vi "Update Command.vi"(6 "Time":dbl, 8 "error in (no error)":errorcluster, 11 "2WayValve in":refnum<class "2WayValveH.lvclass">) -> (0 "error out":errorcluster, 3 "2WayValve out":refnum<class "2WayValveH.lvclass">)   [LabVIEW 2020, in "VolatusGUIElements.lvlib" / "2WayValveH.lvclass"]
uses:
  2WayValveH.lvclass
  2WayValveH.lvclass/2WayValveH.ctl
  lv-vecto/Vecto/Channel/Channel.lvclass/Channel.ctl
  lv-vecto/Vecto/Group/Value by Index.vi
  lv-vecto/Vecto/Channel/Channel.lvclass
  lv-vecto/Vecto/Vecto.lvlib
  VolatusGUIElements.lvlib
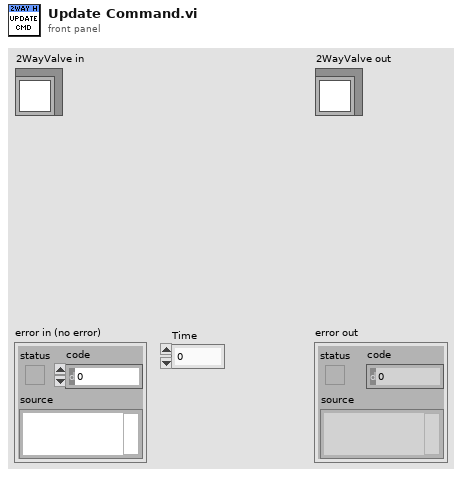
[diagram p1: front panel]
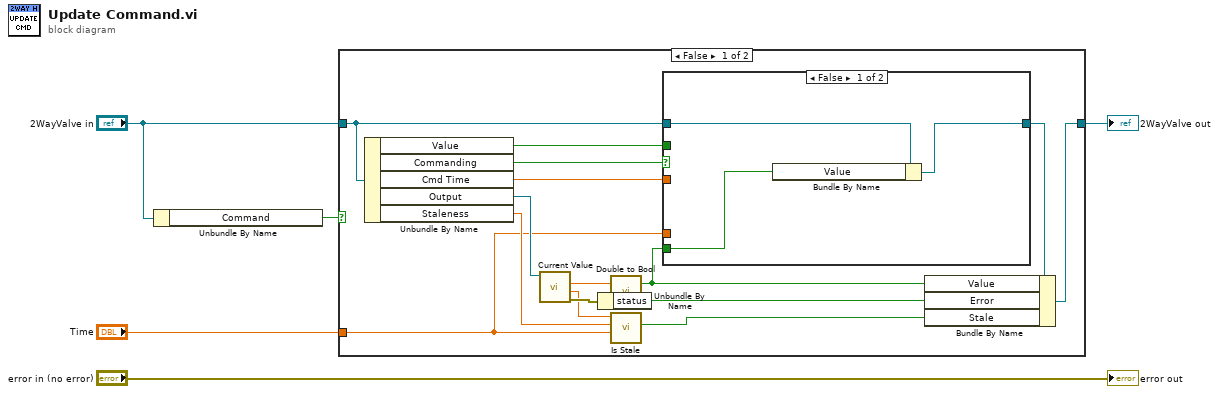
[diagram p0: block diagram]
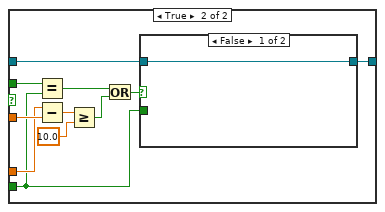
[diagram p2: hidden frame]
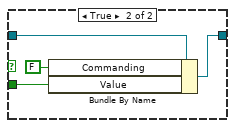
[diagram p3: hidden frame]
diagram:
  n1 = Unbundle By Name("2WayValve in") -> ("Command"=w4:bool)
  n2 = case shown="False" w4 {
    tunnel: [w16 w40] -> w3
    tunnel: "2WayValve in" -> [w12 w40]
    tunnel: "Time" -> [w7 _]
    frame False {
      n3 = Unbundle By Name(w12) -> ("Value"=w13:bool, "Commanding"=w15:bool, "Cmd Time"=w14:dbl, "Output"=w19:refnum<class "Channel.lvclass">, "Staleness"=w8:dbl)
      n4 = call "Current Value.vi"("Channel in"=w19) -> ("error out"=w20:errorcluster, "Timestamp"=w9:dbl, "Scaled"=w18:dbl)  [unwired: 6 in, 2 out]
      n5 = Unbundle By Name(w20) -> ("status"=w17:bool)
      n6 = call "Double to Bool.vi"("Double"=w18) -> ("Bool"=w11:bool)  [unwired: 2 in]
      n7 = call "Is Stale.vi"("Time"=w7, "Staleness"=w8, "Timestamp"=w9) -> ("Stale"=w6:bool)  [unwired: 8 in]
      n8 = case shown="False" w15 {
        tunnel: w14 -> [_ w34]
        tunnel: w13 -> [_ w32]
        tunnel: w7 -> [_ w33]
        tunnel: w12 -> [w23 w27]
        tunnel: w11 -> [w21 w24]
        tunnel: [w22 w26] -> w10
        frame False {
          n9 = Bundle By Name(cluster=w23, "Value"=w21) -> (w22:refnum<class "2WayValveH.lvclass">)
        }
        frame True {
          n10 = Equal?(x=w32, y=w24) -> (x = y?=w31:bool)
          n11 = Subtract(x=w33, y=w34) -> (x-y=w30:dbl)
          n12 = Greater Or Equal?(x=w30, y=10.0) -> (x >= y?=w28:bool)
          n13 = Or(x=w31, y=w28) -> (x .or. y?=w25:bool)
          n14 = case shown="False" w25 {
            tunnel: w27 -> [w35 w39]
            tunnel: [w35 w38] -> w26
            tunnel: w24 -> [_ w36]
            frame False {
            }
            frame True {
              n15 = Bundle By Name(cluster=w39, "Commanding"=FALSE, "Value"=w36) -> (w38:refnum<class "2WayValveH.lvclass">)
            }
          }
        }
      }
      n16 = Bundle By Name(cluster=w10, "Value"=w11, "Error"=w17, "Stale"=w6) -> (w16:refnum<class "2WayValveH.lvclass">)
    }
    frame True {
      # "Command Unused"
    }
  }
  "2WayValve out" <- w3
  "error out" <- "error in (no error)"
